vi "选择性通道波形显示.vi"(0 "布尔":bool, 1 "布尔 2":bool, 2 "振动信号":waveform(dbl)[](graph), 3 "布尔 3":bool, 4 "布尔 4":bool) -> (7 "选择性显示通道信号":waveform(dbl)[](graph))   [LabVIEW 2014]
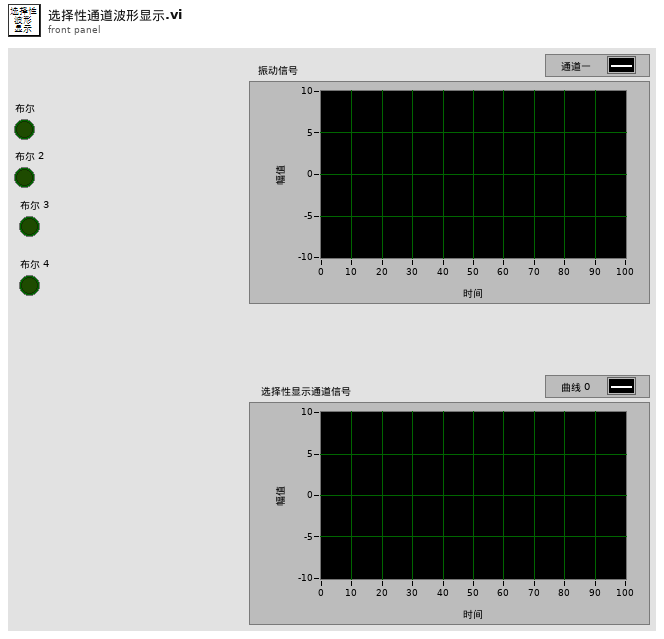
[diagram p1: front panel]
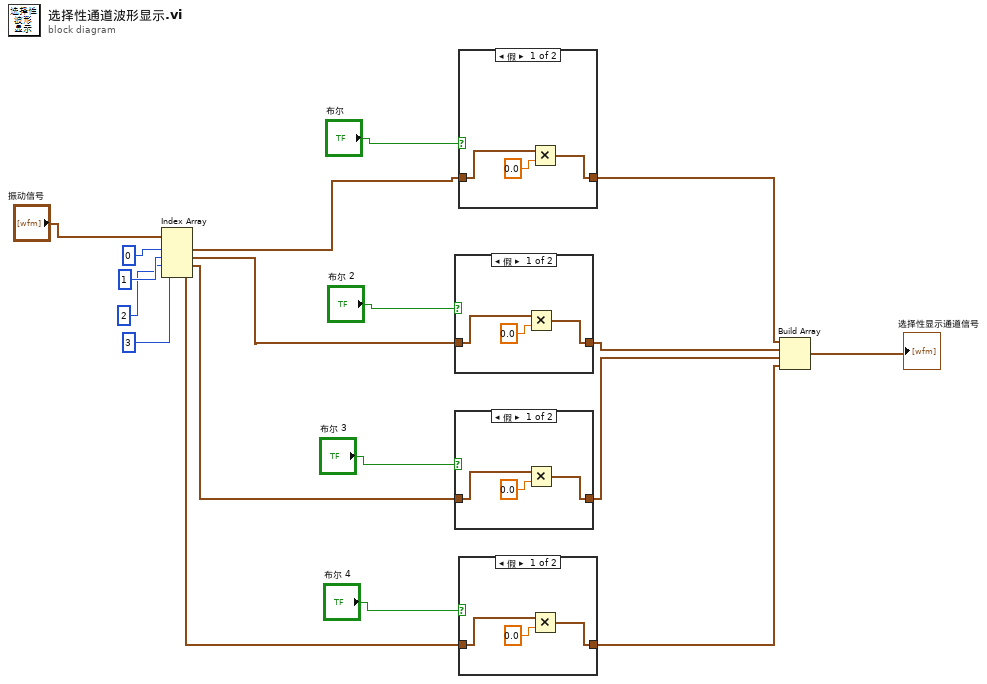
[diagram p0: block diagram]
diagram:
  n1 = Index Array(array="振动信号", index #1=0, index #2=1, index #3=2, index #4=3) -> (element #1=w12:waveform(dbl), element #2=w10:waveform(dbl), element #3=w8:waveform(dbl), element #4=w6:waveform(dbl))
  n2 = case shown="假" "布尔 2" {
    tunnel: w10 -> [w21 w22]
    tunnel: [w19 w22] -> w5
    frame False {
      n3 = Multiply(x=w21, y=0.0) -> (x*y=w19:waveform(dbl))
    }
    frame True {
    }
  }
  n4 = case shown="假" "布尔 3" {
    tunnel: w8 -> [w25 w26]
    tunnel: [w23 w26] -> w4
    frame False {
      n5 = Multiply(x=w25, y=0.0) -> (x*y=w23:waveform(dbl))
    }
    frame True {
    }
  }
  n6 = case shown="假" "布尔" {
    tunnel: w12 -> [w29 w30]
    tunnel: [w27 w30] -> w1
    frame False {
      n7 = Multiply(x=w29, y=0.0) -> (x*y=w27:waveform(dbl))
    }
    frame True {
    }
  }
  n8 = case shown="假" "布尔 4" {
    tunnel: w6 -> [w33 w34]
    tunnel: [w31 w34] -> w3
    frame False {
      n9 = Multiply(x=w33, y=0.0) -> (x*y=w31:waveform(dbl))
    }
    frame True {
    }
  }
  n10 = Build Array(w1, w5, w4, w3) -> (→"选择性显示通道信号":waveform(dbl)[])
